vi "Has Enough Bytes.vi"(1 "required":i32, 2 "ByteArrayTuple in":refnum<class "Bytestream.lvclass">) -> (0 "enough?":bool)   [LabVIEW 2020, in "NI_Bytestream.lvlib" / "Bytestream.lvclass"]
uses:
  <vilib>/Array/Bytestream/Bytestream.lvclass
  <vilib>/Array/Bytestream/Bytestream.lvclass/Bytestream.ctl
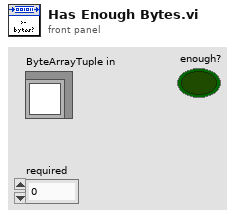
[diagram p1: front panel]
types:
  T1 = typedef "NI_Bytestream.lvlib/Bytestream.lvclass/Datum.ctl" = cluster{"array":u8[], "index":i32}
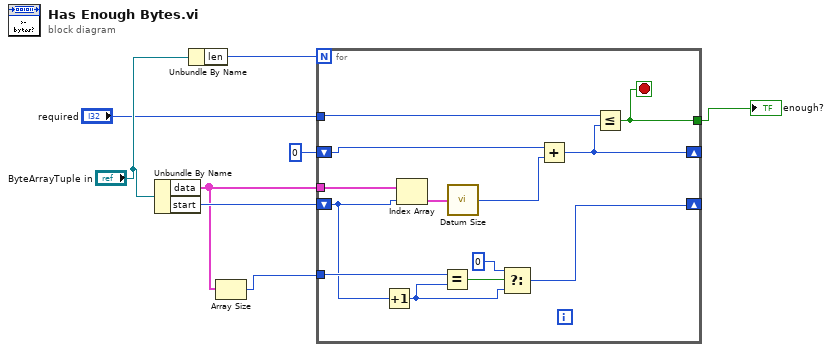
[diagram p0: block diagram]
diagram:
  n1 = Unbundle By Name("ByteArrayTuple in") -> ("data"=w4:T1[], "start"=w5:i32)
  n2 = Unbundle By Name("ByteArrayTuple in") -> ("len"=w7:i32)
  n3 = Array Size(array=w4) -> (size(s)=w3:i32)
  n4 = for {
    N: w7 -> [_]
    shift-right: [w10] -> _
    shift-left: 0 -> [w21]
    tunnel: w4 -> [w15]
    shift-right: [w16] -> _
    shift-left: w5 -> [w14]
    tunnel: w3 -> [w17]
    tunnel: "required" -> [w11]
    tunnel: [w9] -> w1
    stop <- w9 stop-if-true
    n5 = Increment(x=w14) -> (x+1=w19:i32)
    n6 = Index Array(array=w15, index=w14) -> (element=w13:T1)
    n7 = Equal?(x=w17, y=w19) -> (x = y?=w20:bool)
    n8 = call <vilib>:"Datum Size.vi"("datum"=w13) -> ("size"=w12:i32)
    n9 = Select(t=0, s=w20, f=w19) -> (s? t:f=w16:i32)
    n10 = Add(x=w21, y=w12) -> (x+y=w10:i32)
    n11 = Less Or Equal?(x=w11, y=w10) -> (x <= y?=w9:bool)
  }
  "enough?" <- w1
